vi "Connection State Callback Type.vi"(7 "Owner":refnum<class>, 8 "error in (no error)":errorcluster, 10 "Connection State":T1, 11 "Connection":refnum<class "Connection.lvclass">) -> (0 "error out":errorcluster)   [LabVIEW 2020, in "Stream.lvlib"]
uses:
  Stream.lvlib
  Connection/Connection.lvclass
  Connection State.ctl
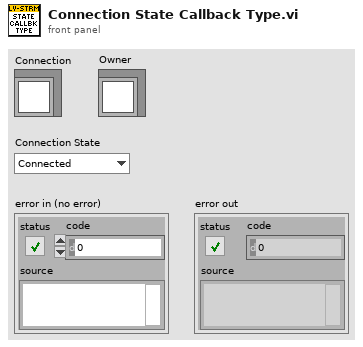
[diagram p1: front panel]
types:
  T1 = typedef "Stream.lvlib/Connection State.ctl" = enum16{"Connected", "Disconnected"}
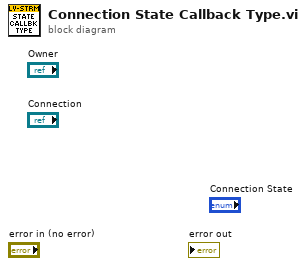
[diagram p0: block diagram]
diagram:
